vi "转换-日期字符串至数值时间数组.vi"(9 "分隔符（/）":string="/", 11 "日期时间（或仅日期）字符串":string) -> (0 "年月日数组":i32[](array[numeric]), 1 "D":i32, 2 "M":i32, 3 "Y":i32, 5 "时间标识":timestamp)   [LabVIEW 2017]
doc: "时间日期字符串转换为 时间标识"
uses:
  <vilib>/Utility/miscctls.llb/LVDateTimeRec.ctl
panel:
  out "秒":i32
  out "分":i32
  out "时":i32
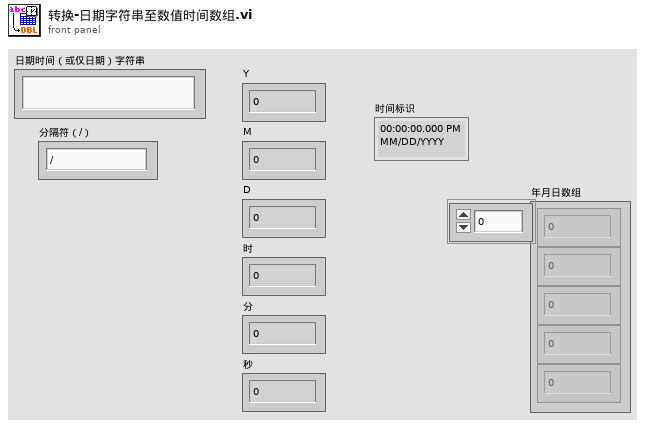
[diagram p1: front panel]
types:
  T1 = typedef "LVDateTimeRec.ctl" = cluster{"fractional second":dbl, "second":i32, "minute":i32, "hour":i32, "day of month":i32, "month":i32, "year":i32, "day of week":i32, "day of year":i32, "DST":i32}
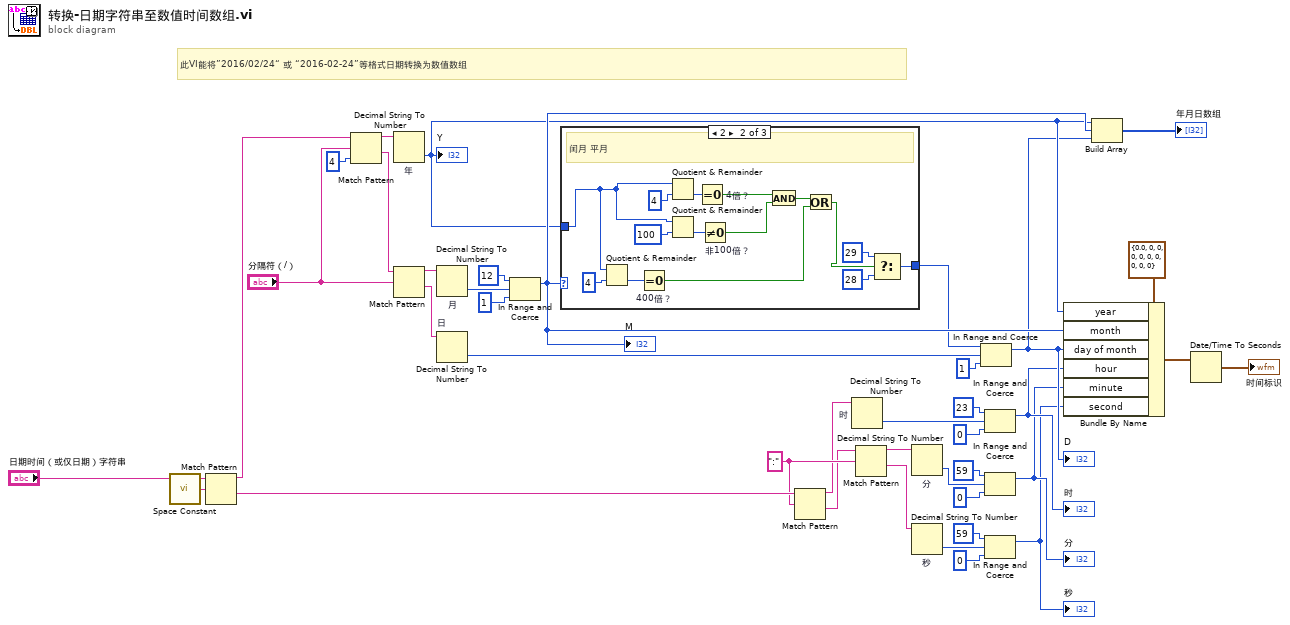
[diagram p0: block diagram]
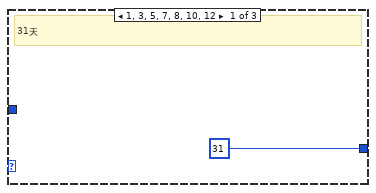
[diagram p2: hidden frame]
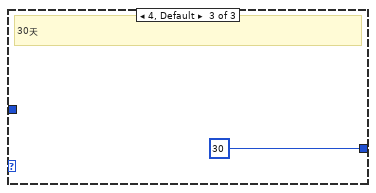
[diagram p3: hidden frame]
diagram:
  w26 = ":" ("正则表达式")
  # "此VI能将”2016/02/24“ 或 “2016-02-24”等格式日期转换为数值数组"
  n1 = call <vilib>:"Space Constant.vi"() -> ("String"=w29:string)
  n2 = Match Pattern(string="日期时间（或仅日期）字符串", regular expression=w29) -> (before substring=w28:string, after substring=w27:string)  [unwired: 1 in, 2 out]
  n3 = Match Pattern(string=w28, regular expression="分隔符（/）", offset (0)=4 ("偏移量(0)")) -> (before substring=w38:string, after substring=w39:string)  [unwired: 2 out]
  n4 = Decimal String To Number "年"(string=w38) -> (number=w16:i32)  [unwired: 2 in, 1 out]
  "Y" <- w16
  n5 = Match Pattern(string=w39, regular expression="分隔符（/）") -> (before substring=w37:string, after substring=w36:string)  [unwired: 1 in, 2 out]
  n6 = Decimal String To Number "月"(string=w37) -> (number=w21:i32)  [unwired: 2 in, 1 out]
  n7 = Decimal String To Number "日"(string=w36) -> (number=w18:i32)  [unwired: 2 in, 1 out]
  n8 = In Range and Coerce(upper limit=12 ("上限"), x=w21, lower limit=1 ("上限")) -> (coerced(x)=w17:i32)  [unwired: 1 out]
  "M" <- w17
  n9 = case shown="2" w17 {
    tunnel: w16 -> [_ w42 _]
    tunnel: [31 ("y") w54 30 ("y")] -> w15
    frame 1, 3, 5, 7, 8, 10, 12 {
      # "31天"
    }
    frame 2 {
      # "闰月 平月"
      n10 = Quotient & Remainder(x=w42, y=u16 4) -> (floor(x/y)=w47:i32)  [unwired: 1 out]
      n11 = Equal To 0? "400倍？"(x=w47) -> (x = 0?=w53:bool)
      n12 = Quotient & Remainder(x=w42, y=u16 4) -> (floor(x/y)=w45:i32)  [unwired: 1 out]
      n13 = Quotient & Remainder(x=w42, y=u16 100) -> (floor(x/y)=w50:i32)  [unwired: 1 out]
      n14 = Equal To 0? "4倍？"(x=w45) -> (x = 0?=w46:bool)
      n15 = Not Equal To 0? "非100倍？"(x=w50) -> (x != 0?=w52:bool)
      n16 = And(x=w46, y=w52) -> (x .and. y?=w51:bool)
      n17 = Or(x=w51, y=w53) -> (x .or. y?=w43:bool)
      n18 = Select(t=29 ("y"), s=w43, f=28 ("y")) -> (s? t:f=w54:i32)
    }
    frame 4, Default {
      # "30天"
    }
  }
  n19 = Match Pattern(string=w27, regular expression=w26) -> (before substring=w24:string, after substring=w25:string)  [unwired: 1 in, 2 out]
  n20 = Decimal String To Number "时"(string=w24) -> (number=w12:i32)  [unwired: 2 in, 1 out]
  n21 = Match Pattern(string=w25, regular expression=w26) -> (before substring=w23:string, after substring=w22:string)  [unwired: 1 in, 2 out]
  n22 = Decimal String To Number "分"(string=w23) -> (number=w8:i32)  [unwired: 2 in, 1 out]
  n23 = Decimal String To Number "秒"(string=w22) -> (number=w4:i32)  [unwired: 2 in, 1 out]
  n24 = In Range and Coerce(upper limit=w15, x=w18, lower limit=1 ("上限")) -> (coerced(x)=w13:i32)  [unwired: 1 out]
  "D" <- w13
  n25 = In Range and Coerce(upper limit=23 ("上限"), x=w12, lower limit=0 ("下限")) -> (coerced(x)=w9:i32)  [unwired: 1 out]
  "时" <- w9
  n26 = In Range and Coerce(upper limit=59 ("上限"), x=w8, lower limit=0 ("下限")) -> (coerced(x)=w5:i32)  [unwired: 1 out]
  "分" <- w5
  n27 = In Range and Coerce(upper limit=59 ("上限"), x=w4, lower limit=0 ("下限")) -> (coerced(x)=w1:i32)  [unwired: 1 out]
  "秒" <- w1
  n28 = Bundle By Name(cluster=T1 {"fractional second"=0.0, "second"=0, "minute"=0, "hour"=0, "day of month"=0, "month"=0, "year"=0, "day of week"=0, "day of year"=0, "DST"=0} ("日期时间记录"), "year"=w16, "month"=w17, "day of month"=w13, "hour"=w9, "minute"=w5, "second"=w1) -> (w32:T1)
  n29 = Build Array(w16, w17, w13) -> (→"年月日数组":i32[])
  n30 = Date/Time To Seconds(2:w32) -> (0:→"时间标识":timestamp)  [unwired: 1 in]
